vi "FPGA_CounterWriteReset.vi"(8 "error in (no error)":errorcluster, 11 "Ctr Ref in":T1={"DevStatus"={"status"=FALSE, "code"=0, "source"=""}, "CntIndex"=enum."Ctr 1"}) -> (0 "error out":errorcluster, 3 "Ctr Ref out":T1={"DevStatus"={"status"=FALSE, "code"=0, "source"=""}, "CntIndex"=enum."Ctr 1"})   [LabVIEW 2017]
uses:
  <vilib>/Rock Robotics/SystemInterfaces/Counter/FPGA_CounterCtrDevRef.ctl
  <vilib>/Rock Robotics/SystemInterfaces/Counter/FPGA_CounterCtrSystemIndex.ctl
  <vilib>/Rock Robotics/SystemInterfaces/System/FPGA_SystemFPGA Ref Global.vi
  <vilib>/Utility/error.llb/Error Cluster From Error Code.vi
  <vilib>/rvi/errors/niLvFpgaAdjustHostInterfaceError.vi
  <vilib>/rvi/interface/nirviReadWriteControl/nirviReadWriteControl.xnode
  <vilib>/Rock Robotics/SystemInterfaces/System/FPGA_SystemFRC FPGA Ref.ctl
  NiFpgaLv.dll
  <vilib>/rvi/interface/Simulation/niFpgaSimulationCallBeginRW.vi
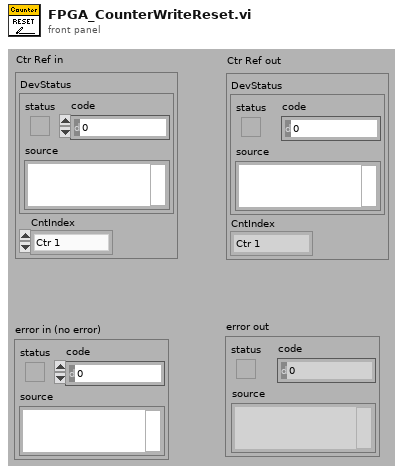
[diagram p1: front panel]
types:
  T1 = typedef "FPGA_CounterCtrDevRef.ctl" = cluster{"DevStatus":errorcluster, "CntIndex":T2}
  T2 = typedef "FPGA_CounterCtrSystemIndex.ctl" = enum8{"Ctr 0", "Ctr 1", "Ctr 2", "Ctr 3", "Ctr 4", "Ctr 5", "Ctr 6", "Ctr 7", "Invalid"}
  T3 = typedef "FPGA_SystemFRC FPGA Ref.ctl" = refnum<k20>
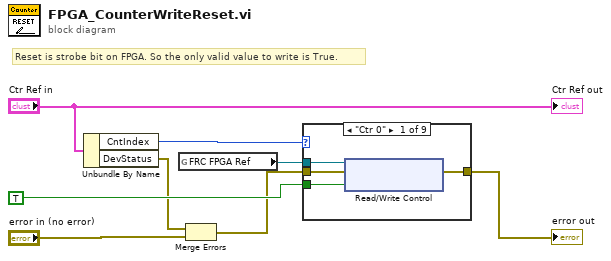
[diagram p0: block diagram]
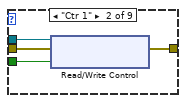
[diagram p2: hidden frame]
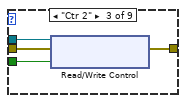
[diagram p3: hidden frame]
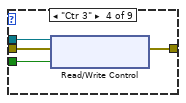
[diagram p4: hidden frame]
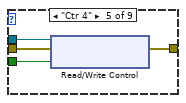
[diagram p5: hidden frame]
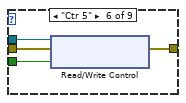
[diagram p6: hidden frame]
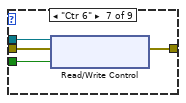
[diagram p7: hidden frame]
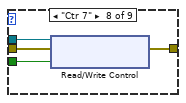
[diagram p8: hidden frame]
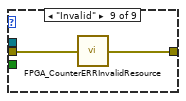
[diagram p9: hidden frame]
diagram:
  # "Reset is strobe bit on FPGA. So the only valid value to write is True."
  n1 = Unbundle By Name("Ctr Ref in") -> ("CntIndex"=w6:T2, "DevStatus"=w4:errorcluster)
  n2 = global read "FPGA_SystemFPGA Ref Global.vi" "FRC FPGA Ref"() -> (w2:T3)
  n3 = Merge Errors(w4, "error in (no error)") -> (w3:errorcluster)
  n4 = case shown="\"Ctr 0\"" w6 {
    tunnel: w2 -> [w11 w16 w20 w24 w28 w32 w36 w40 _]
    tunnel: w3 -> [w12 w15 w19 w23 w27 w31 w35 w39 w42]
    tunnel: [w10 w14 w18 w22 w26 w30 w34 w38 w41] -> w7
    tunnel: TRUE ("Reset") -> [w9 w13 w17 w21 w25 w29 w33 w37 _]
    frame "Ctr 0" {
      n5 = xnode "Read/Write Control"("FPGA VI Reference In"=w11, "error in"=w12, "Counter0.Reset"=w9) -> ("error out"=w10:errorcluster)  [unwired: 1 out]
    }
    frame "Ctr 1" {
      n6 = xnode "Read/Write Control"("FPGA VI Reference In"=w16, "error in"=w15, "Counter1.Reset"=w13) -> ("error out"=w14:errorcluster)  [unwired: 1 out]
    }
    frame "Ctr 2" {
      n7 = xnode "Read/Write Control"("FPGA VI Reference In"=w20, "error in"=w19, "Counter2.Reset"=w17) -> ("error out"=w18:errorcluster)  [unwired: 1 out]
    }
    frame "Ctr 3" {
      n8 = xnode "Read/Write Control"("FPGA VI Reference In"=w24, "error in"=w23, "Counter3.Reset"=w21) -> ("error out"=w22:errorcluster)  [unwired: 1 out]
    }
    frame "Ctr 4" {
      n9 = xnode "Read/Write Control"("FPGA VI Reference In"=w28, "error in"=w27, "Counter4.Reset"=w25) -> ("error out"=w26:errorcluster)  [unwired: 1 out]
    }
    frame "Ctr 5" {
      n10 = xnode "Read/Write Control"("FPGA VI Reference In"=w32, "error in"=w31, "Counter5.Reset"=w29) -> ("error out"=w30:errorcluster)  [unwired: 1 out]
    }
    frame "Ctr 6" {
      n11 = xnode "Read/Write Control"("FPGA VI Reference In"=w36, "error in"=w35, "Counter6.Reset"=w33) -> ("error out"=w34:errorcluster)  [unwired: 1 out]
    }
    frame "Ctr 7" {
      n12 = xnode "Read/Write Control"("FPGA VI Reference In"=w40, "error in"=w39, "Counter7.Reset"=w37) -> ("error out"=w38:errorcluster)  [unwired: 1 out]
    }
    frame "Invalid" {
      n13 = call <vilib>:"FPGA_CounterERRInvalidResource.vi"("error in (no error)"=w42) -> ("error out"=w41:errorcluster)
    }
  }
  "error out" <- w7
  "Ctr Ref out" <- "Ctr Ref in"
